vi "waveform list.vi"() -> ()   [LabVIEW 2018]
panel:
  out "波形图表":waveform(dbl)[](graph)
  out "布尔 2":bool
  out "布尔":bool
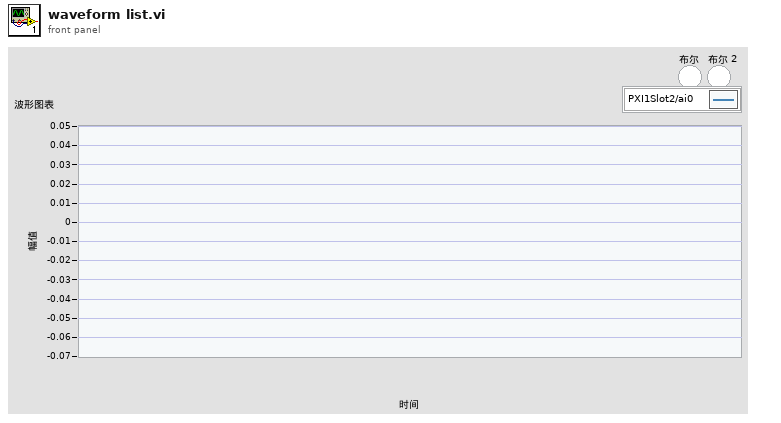
[diagram p1: front panel]
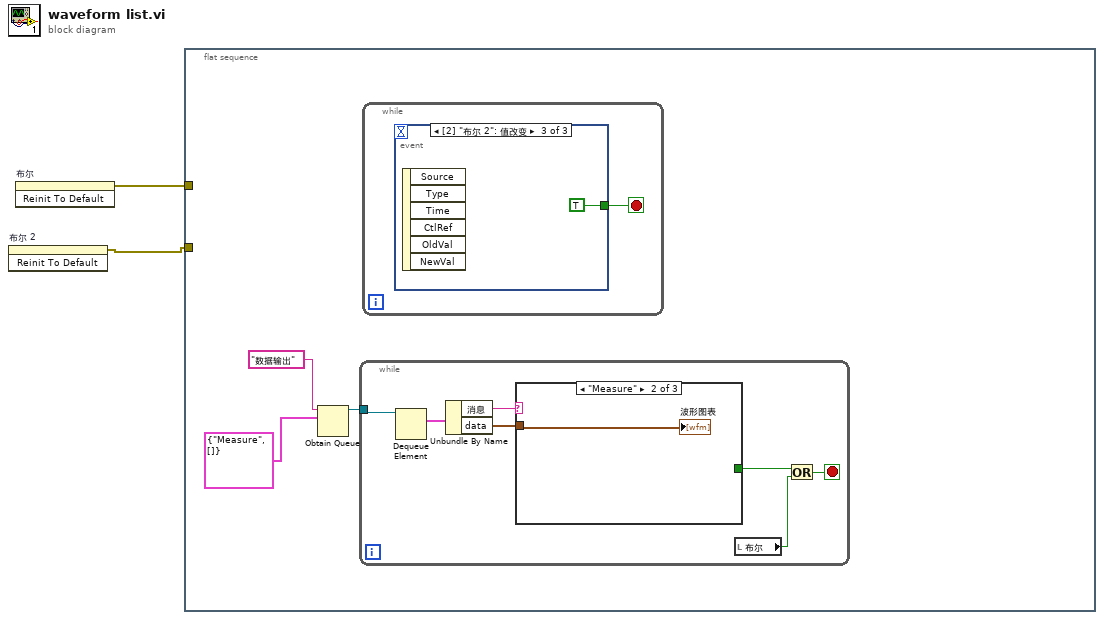
[diagram p0: block diagram]
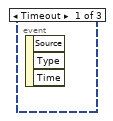
[diagram p2: hidden frame]
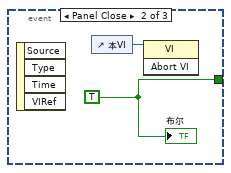
[diagram p3: hidden frame]
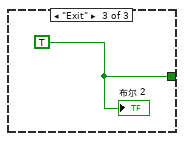
[diagram p5: hidden frame]
diagram:
  n1 = invoke on="布尔 2" class="Bool (严格)" method="Reinit To Default"() -> (error out=w1:errorcluster)  [unwired: 3 in, 2 out]
  n2 = invoke on="布尔" class="Bool (严格)" method="Reinit To Default"() -> (error out=w2:errorcluster)  [unwired: 3 in, 2 out]
  n3 = flat-sequence {
    tunnel: w2 -> [_]
    tunnel: w1 -> [_]
    frame #0 {
      n4 = Obtain Queue(name (unnamed)="数据输出" ("名称（未命名）"), element data type=cluster{"消息":string, "data":waveform(dbl)[]} {"消息"="Measure", "data"=[]}) -> (queue out=w4:refnum<queue>)  [unwired: 3 in, 2 out]
      n5 = while {
        tunnel: w4 -> [w12]
        stop <- w14 stop-if-true
        n6 = Dequeue Element(queue=w12) -> (element=w11:cluster{"消息":string, "data":waveform(dbl)[]})  [unwired: 2 in, 3 out]
        n7 = Unbundle By Name(w11) -> ("消息"=w10:string, "data"=w13:waveform(dbl)[])
        n8 = case shown="\"Measure\"" w10 {
          tunnel: [_ _ w18] -> w15
          tunnel: w13 -> [_ w17 _]
          frame "假", Default {
          }
          frame "Measure" {
            "波形图表" <- w17
          }
          frame "Exit" {
            w18 = TRUE
            "布尔 2" <- w18
          }
        }
        n9 = local read "布尔"() -> (w16:bool)
        n10 = Or(x=w15, y=w16) -> (x .or. y?=w14:bool)
      }
      n11 = while {
        stop <- w6 stop-if-true
        n12 = event shown="[2] \"布尔 2\": 值改变" {
          selector: _ -> [_ _ _]
          dyn-events: _ -> [_ _ _]
          timeout: _ -> [_ _ _]
          tunnel: [_ w8 TRUE] -> w6
          event Timeout {
            n13 = event-data() -> ()  [unwired: 1 in, 3 out]
          }
          event Panel Close {
            w8 = TRUE
            n14 = event-data() -> ()  [unwired: 1 in, 4 out]
            n15 = control-ref of="本VI"() -> (w7:refnum<vi>)
            n16 = invoke class="VI" method="Abort VI"(reference=w7) -> ()  [unwired: 2 in, 3 out]
            "布尔" <- w8
          }
          event "布尔 2": Value Change {
            n17 = event-data() -> ()  [unwired: 1 in, 6 out]
          }
        }
      }
    }
  }
